vi "process position.vi"(5 "Fs reading":dbl, 6 "Gyro LSB":dbl, 7 "Gyro %":dbl, 8 "Gyro data":cluster{"Gyro X LSB":i16, "Gyro Y LSB":i16}, 9 "Acc pos":cluster{"X acc":dbl, "Y acc":dbl}, 11 "Pos cluster ref":refnum<vi>) -> ()   [LabVIEW 2017]
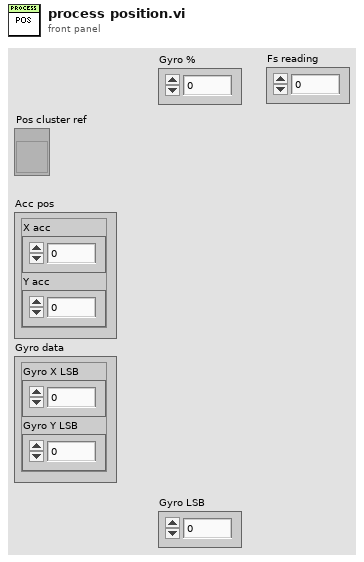
[diagram p1: front panel]
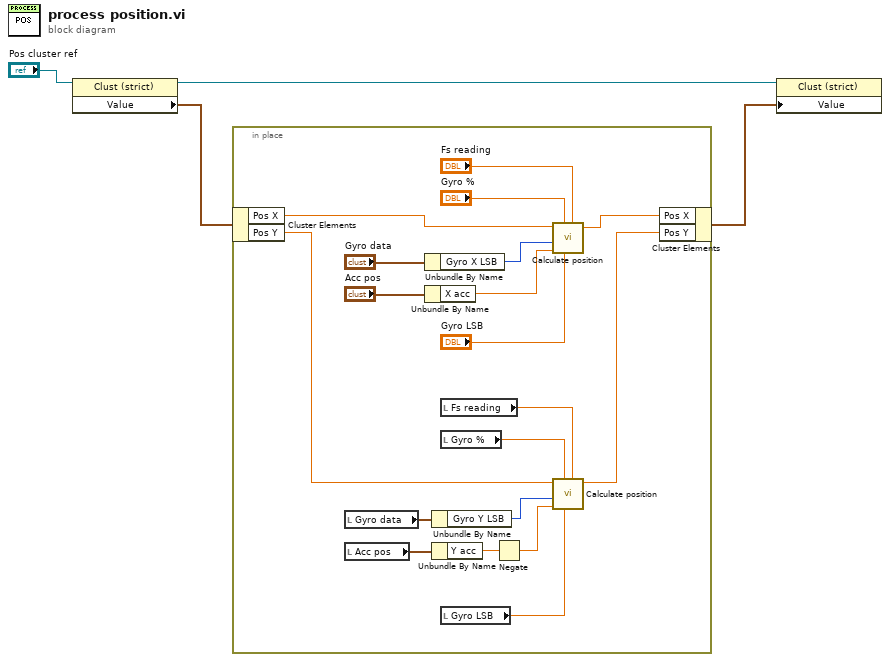
[diagram p0: block diagram]
diagram:
  n1 = property class="Clust (strict)"(reference="Pos cluster ref") -> (reference out=w3:refnum<vi>, "Value"=w2:cluster{"Pos X":dbl, "Pos Y":dbl, "Pos Z":dbl})  [unwired: 1 in, 1 out]
  n2 = in-place {
    n3 = in-place-cluster #1(w2) -> ("Pos X"=w21:dbl, "Pos Y"=w16:dbl)
    n4 = local read "Gyro data"() -> (w9:cluster{"Gyro X LSB":i16, "Gyro Y LSB":i16})
    n5 = local read "Acc pos"() -> (w8:cluster{"X acc":dbl, "Y acc":dbl})
    n6 = Unbundle By Name("Gyro data") -> ("Gyro X LSB"=w10:i16)
    n7 = Unbundle By Name("Acc pos") -> ("X acc"=w12:dbl)
    n8 = Unbundle By Name(w9) -> ("Gyro Y LSB"=w6:i16)
    n9 = Unbundle By Name(w8) -> ("Y acc"=w5:dbl)
    n10 = local read "Fs reading"() -> (w17:dbl)
    n11 = local read "Gyro %"() -> (w15:dbl)
    n12 = local read "Gyro LSB"() -> (w14:dbl)
    n13 = Negate(x=w5) -> (-x=w7:dbl)
    n14 = call "Calculate position.vi"("Fs reading"="Fs reading", "Gyro LSB"="Gyro LSB", "Gyro %"="Gyro %", "Acc position (radians)"=w12, "Gyro position (LSB)"=w10, "Old position"=w21) -> ("New position"=w22:dbl)  [unwired: 5 in]
    n15 = call "Calculate position.vi"("Fs reading"=w17, "Gyro LSB"=w14, "Gyro %"=w15, "Acc position (radians)"=w7, "Gyro position (LSB)"=w6, "Old position"=w16) -> ("New position"=w23:dbl)  [unwired: 5 in]
    n16 = in-place-cluster #1("Pos X"=w22, "Pos Y"=w23) -> (w4:cluster{"Pos X":dbl, "Pos Y":dbl, "Pos Z":dbl})
  }
  n17 = property class="Clust (strict)"(reference=w3, "Value"=w4) -> ()  [unwired: 1 in, 2 out]
